vi "AT Clear All Buffers A.vi"(8 "error in (no error)":errorcluster, 11 "Handle":u32) -> (0 "error out":errorcluster, 3 "Status":i32)   [LabVIEW 2019]
doc: "Clear All Buffers\n\nOutput:\n I32 Status \n\nInput:\n I32 Handle\n\nDeletes any buffers that have been created but not yet deleted."
uses:
  atcoreA.dll
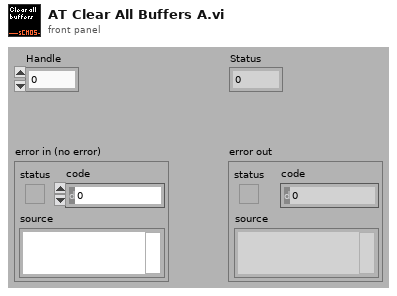
[diagram p1: front panel]
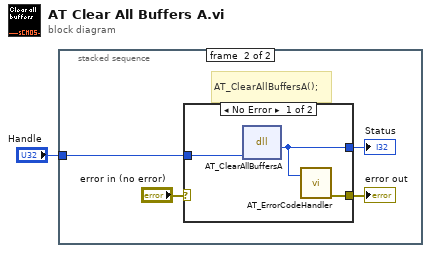
[diagram p0: block diagram]
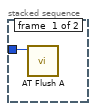
[diagram p2: hidden frame]
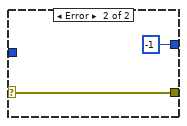
[diagram p3: hidden frame]
diagram:
  n1 = stacked-sequence {
    tunnel: "Handle" -> [w2 w3]
    frame #0 {
      n2 = call <userlib>:"AT Flush A.vi"("Handle"=w2) -> ()  [unwired: 9 in, 2 out]
    }
    frame #1 {
      # "AT_ClearAllBuffersA();"
      n3 = case shown="No Error" "error in (no error)" {
        selector: "error in (no error)" -> [_ w11]
        tunnel: [w7 -1] -> w4
        tunnel: [w8 w11] -> w6
        tunnel: w3 -> [w9 _]
        frame No Error {
          n4 = dll-call lib="atcoreA.dll" fn="AT_ClearAllBuffersA"("Handle"=w9) -> ("Status"=w7:i32)  [unwired: 4 in, 2 out]
          n5 = call <userlib>:"AT_ErrorCodeHandler.vi"("Error"=w7) -> ("error out"=w8:errorcluster)  [unwired: 6 in]
        }
        frame Error {
        }
      }
      "Status" <- w4
      "error out" <- w6
    }
  }
